vi "Device Read (Batch).vi"() -> (3 "Device Read (Batch) string":string)   [LabVIEW 2019]
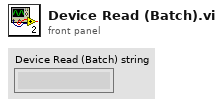
[diagram p1: front panel]
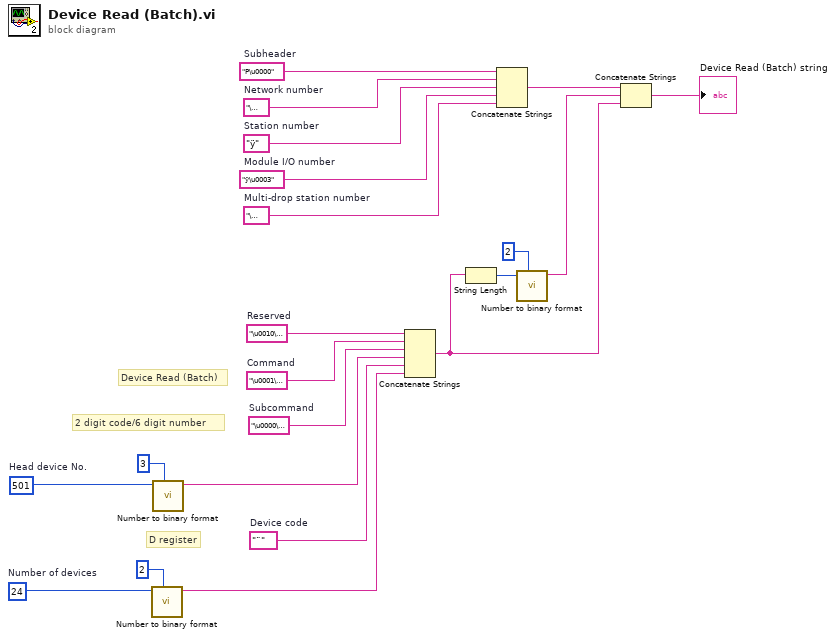
[diagram p0: block diagram]
diagram:
  w14 = u32 24  # Number of devices
  w8 = "¨"  # Device code
  w16 = u32 501  # Head device No.
  w10 = "\u0000\u0000"  # Subcommand
  w11 = "\u0001\u0004"  # Command
  w12 = "\u0010\u0000"  # Reserved
  w17 = "\u0000"  # Multi-drop station number
  w18 = "ÿ\u0003"  # Module I/O number
  w19 = "ÿ"  # Station number
  w20 = "\u0000"  # Network number
  w21 = "P\u0000"  # Subheader
  # "D register"
  # "2 digit code/6 digit number"
  # "Device Read (Batch)"
  n1 = call "Number to binary format.vi"("length in bytes (3)"=2, "Numeric"=w14) -> ("Binary format"=w7:string)  [unwired: 9 in]
  n2 = call "Number to binary format.vi"("length in bytes (3)"=3, "Numeric"=w16) -> ("Binary format"=w9:string)  [unwired: 9 in]
  n3 = Concatenate Strings(w12, w11, w10, w9, w8, w7) -> (w2:string)
  n4 = String Length(string=w2) -> (length=w6:i32)
  n5 = Concatenate Strings(w21, w20, w19, w18, w17) -> (w4:string)
  n6 = call "Number to binary format.vi"("length in bytes (3)"=2, "Numeric"=w6) -> ("Binary format"=w3:string)  [unwired: 9 in]
  n7 = Concatenate Strings(w4, w3, w2) -> (→"Device Read (Batch) string":string)
